vi "UseThisProgramFinal_AlexV1.vi"() -> ()   [LabVIEW 2012]
uses:
  <vilib>/measure/mamon.llb/Trigger Detection for N Channel.vi
  <vilib>/express/express analysis/Spectral/Block/exnSpectralBlock spectral measurements RMS poly.vi
  <vilib>/express/express analysis/Spectral/Block/exnSpectralBlock spectral measurements RMS WFM.vi
  <vilib>/express/express analysis/Spectral/Block/exnSpectralBlock spectral measurements RMS DDT.vi
  <vilib>/express/express analysis/Spectral/XNode/ExpressSpectralMeasurementsBlockNode.xnode
  <vilib>/measure/NI_MAPro.lvlib
panel:
  out "FFT Shifted":cluster{"f0":dbl, "df":dbl, "magnitude":dbl[]}(graph)
  in  "play shifted audio":bool
  in  "autotune on?":bool
  in  "manual frequency \nselection":dbl
  in  "trigger level":dbl[](array[numeric]) format="%0.2f"
  out "Frequency Played":dbl
  out "FFT Original":waveform(dbl)(graph)
  out "Frequency Off By":dbl
  out "Output Frequency":dbl
  out "Note Closest To":string
  out "Shifted Waveform":waveform(dbl)(graph)
  out "Original Waveform":dynamicdata(graph)
  # "yea"
  # "nay"
  # "detect when pluck string, add digital effects, analog switch/potentiometer, playing a song would be awesome"
  # "change later"
  # "nay"
  # "yea"
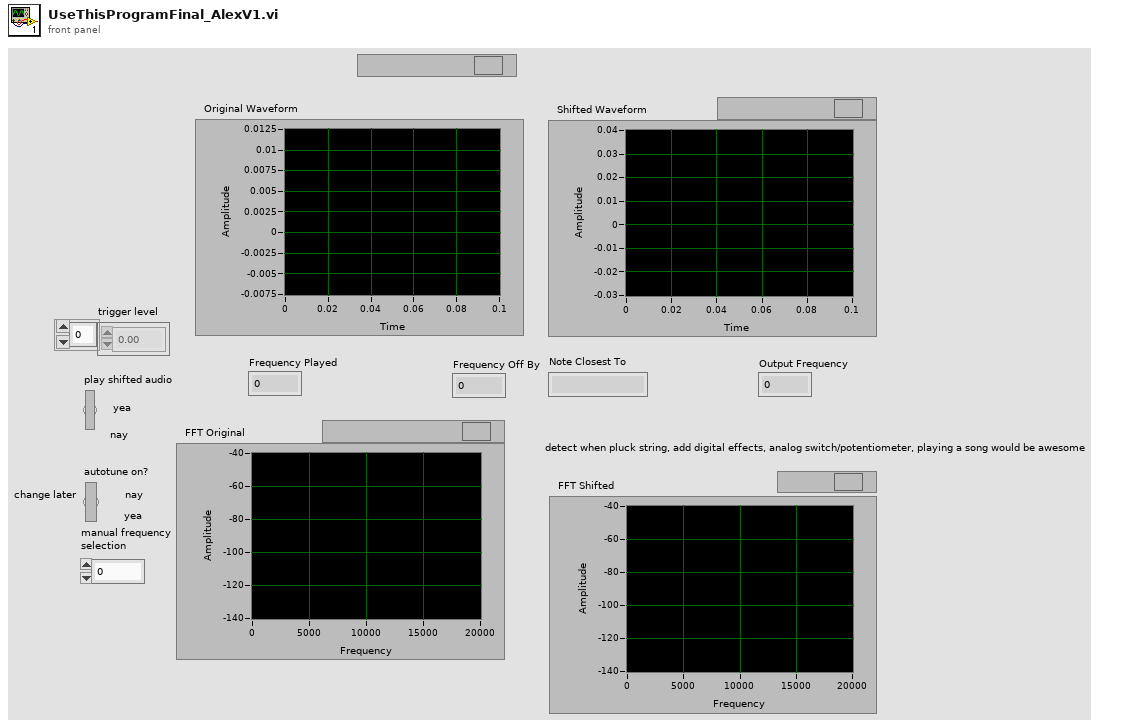
[diagram p1: front panel]
types:
  T1 = cluster{"averaging mode":u16, "weighting mode":u16, "number of averages":u32}
  T2 = cluster{"dB On (F)":bool, "unwrap phase (F)":bool, "convert to degree (F)":bool}
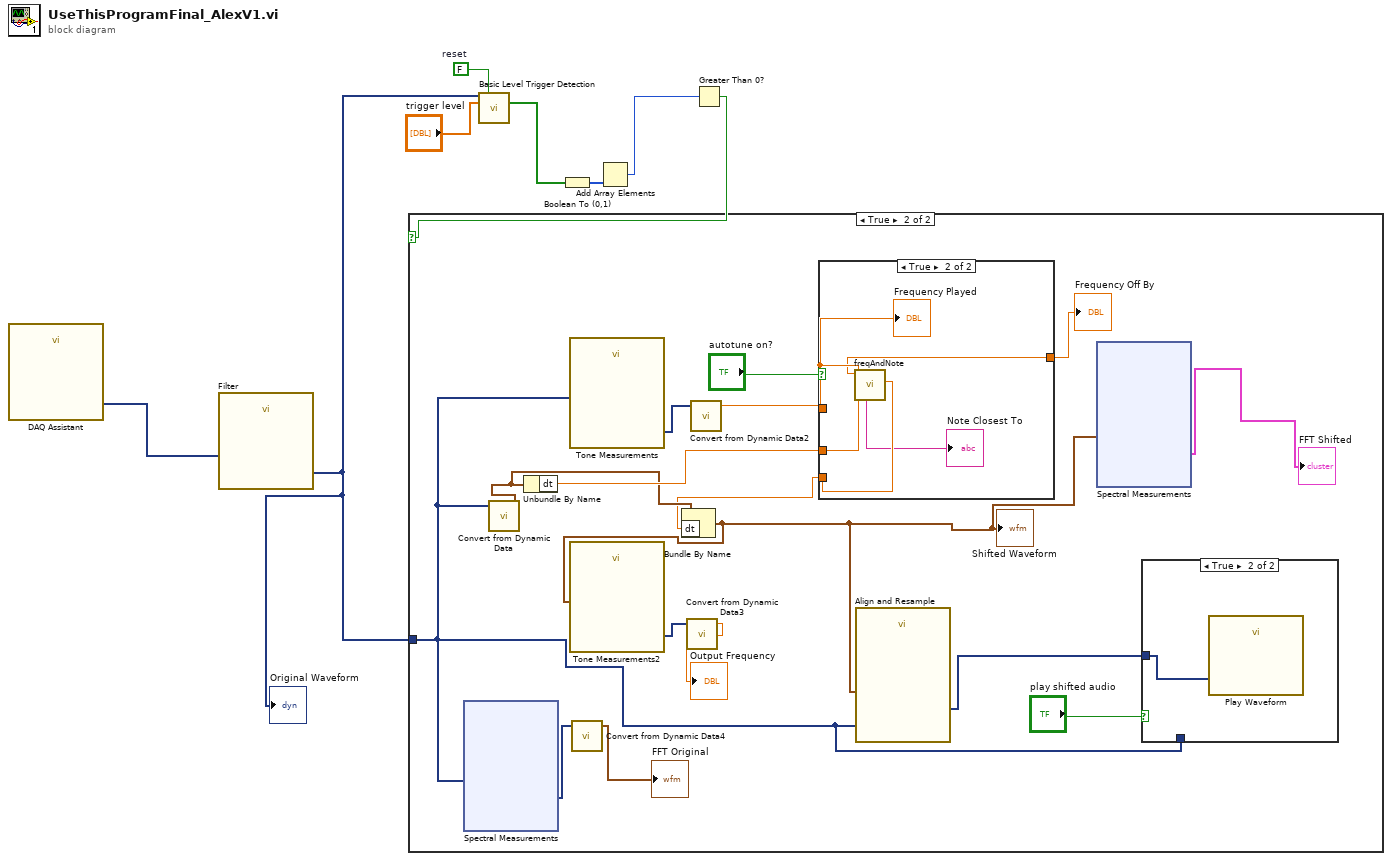
[diagram p0: block diagram]
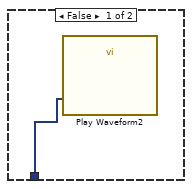
[diagram p3: hidden frame]
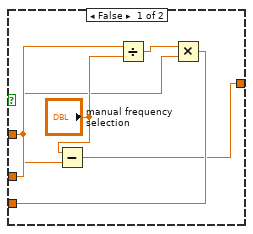
[diagram p4: hidden frame]
diagram:
  w7 = FALSE  # reset
  n1 = call "DAQ Assistant"() -> ("data"=w1:dynamicdata)  [unwired: 17 in, 2 out]
  n2 = call "Filter"("Signal"=w1) -> ("Filtered Signal"=w2:dynamicdata)  [unwired: 9 in, 1 out]
  "Original Waveform" <- w2
  n3 = call-poly <vilib>:"Basic Level Trigger Detection.vi"("signal in"=w2, "reset"=w7, "level"="trigger level") -> ("trigger detected?"=w6:bool[])  [unwired: 10 in, 2 out]
  n4 = Boolean To (0,1)(Boolean=w6) -> (0, 1=w4:i16[])
  n5 = Add Array Elements(numeric array=w4) -> (sum=w3:i16)
  n6 = Greater Than 0?(x=w3) -> (x > 0?=w5:bool)
  n7 = case shown="True" w5 {
    tunnel: w2 -> [_ w13]
    frame False {
    }
    frame True {
      n8 = xnode "Spectral Measurements"("Signals"=w13) -> ("FFT - (RMS)"=w20:dynamicdata)  [unwired: 1 in, 2 out]
      n9 = call "Convert from Dynamic Data"("Dynamic Data Type"=w13) -> ("Waveform"=w18:waveform(dbl))  [unwired: 3 in]
      n10 = Unbundle By Name(w18) -> ("dt"=w24:dbl)
      n11 = call "Tone Measurements"("Signals"=w13) -> ("Frequency"=w23:dynamicdata)  [unwired: 8 in, 2 out]
      n12 = call "Convert from Dynamic Data4"("Dynamic Data Type"=w20) -> ("Waveform"=→"FFT Original":waveform(dbl))  [unwired: 3 in]
      n13 = call "Convert from Dynamic Data2"("Dynamic Data Type"=w23) -> ("Scalar"=w17:dbl)  [unwired: 3 in]
      n14 = case shown="True" "autotune on?" {
        tunnel: w24 -> [w42 w47]
        tunnel: [w40 w46] -> w16
        tunnel: w17 -> [w37 w44]
        tunnel: [w38 w43] -> w9
        frame False {
          n15 = Subtract(x="manual frequency \nselection", y=w37) -> (x-y=w38:dbl)
          n16 = Divide(x=w42, y="manual frequency \nselection") -> (x/y=w41:dbl)
          n17 = Multiply(x=w41, y=w37) -> (x*y=w40:dbl)
        }
        frame True {
          n18 = call "freqAndNote.vi"("dt Original"=w47, "Frequency In"=w44) -> ("output dt"=w46:dbl, "Frequency Off"=w43:dbl, "Note Closest To"=→"Note Closest To":string)  [unwired: 6 in, 1 out]
          "Frequency Played" <- w44
        }
      }
      "Frequency Off By" <- w9
      n19 = Bundle By Name(cluster=w18, "dt"=w16) -> (w11:waveform(dbl))
      "Shifted Waveform" <- w11
      n20 = call "Tone Measurements2"("Signals"=w11) -> ("Frequency"=w22:dynamicdata)  [unwired: 8 in, 2 out]
      n21 = call "Convert from Dynamic Data3"("Dynamic Data Type"=w22) -> ("Scalar"=→"Output Frequency":dbl)  [unwired: 3 in]
      n22 = call "Align and Resample"("Reference Signal"=w13, "Signals"=w11) -> ("Resampled Signals"=w12:dynamicdata)  [unwired: 7 in, 2 out]
      n23 = xnode "Spectral Measurements"("Signals"=w11) -> ("FFT - (RMS)"=→"FFT Shifted":cluster{"f0":dbl, "df":dbl, "magnitude":dbl[]})  [unwired: 1 in, 2 out]
      n24 = case shown="True" "play shifted audio" {
        tunnel: w12 -> [_ w36]
        tunnel: w13 -> [w35 _]
        frame False {
          n25 = call "Play Waveform2"("Data"=w35) -> ()  [unwired: 18 in, 1 out]
        }
        frame True {
          n26 = call "Play Waveform"("Data"=w36) -> ()  [unwired: 18 in, 1 out]
        }
      }
    }
  }
